vi "Set Dependencies.vi"(8 "error in (no error)":errorcluster, 10 "Dependencies":T1, 11 "Instrument in":refnum<class "Instrument.lvclass">) -> (0 "error out":errorcluster, 3 "Instrument out":refnum<class "Instrument.lvclass">)   [LabVIEW 2019, in "Instrument.lvclass"]
uses:
  Instrument.lvclass
  Typedefs/Dependencies--Cluster.ctl
  <userlib>/LevyLab/RemoteControl/RemoteControl.lvclass
  <userlib>/LevyLab/Logger.Error/Logger.Error.lvclass
  <userlib>/LevyLab/Logger.PGSQL/Logger.PGSQL.lvclass
  <userlib>/LevyLab/Configuration/Configuration.lvclass
  subsystems/HAL/HAL.lvclass
  Instrument.lvclass/Instrument.ctl
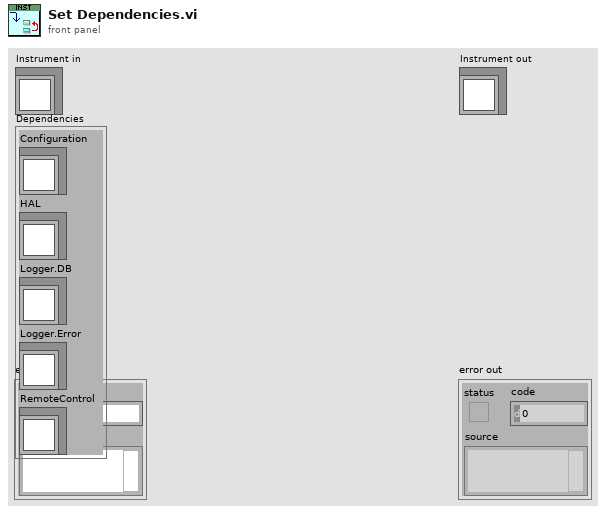
[diagram p1: front panel]
types:
  T1 = typedef "Instrument.lvclass/Dependencies--Cluster.ctl" = cluster{"Configuration":refnum<class "Configuration.lvclass">, "HAL":refnum<class "HAL.lvclass">, "Logger.DB":refnum<class "Logger.PGSQL.lvclass">, "Logger.Error":refnum<class "Logger.Error.lvclass">, "RemoteControl":refnum<class "RemoteControl.lvclass">}
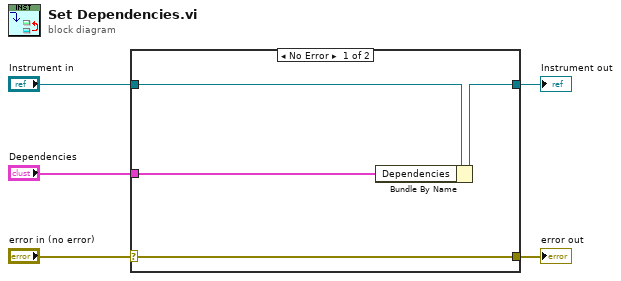
[diagram p0: block diagram]
diagram:
  n1 = case shown="No Error" "error in (no error)" {
    selector: "error in (no error)" -> [w9 w10]
    tunnel: [w9 w10] -> w4
    tunnel: [w7 w11] -> w2
    tunnel: "Instrument in" -> [w8 w11]
    tunnel: "Dependencies" -> [w6 _]
    frame No Error {
      n2 = Bundle By Name(cluster=w8, "Dependencies"=w6) -> (w7:refnum<class "Instrument.lvclass">)
    }
    frame Error {
    }
  }
  "error out" <- w4
  "Instrument out" <- w2
